vi "controlSensorEnabled.vi"(7 "set":bool, 8 "error in":errorcluster, 9 "enableSensor":bool, 10 "axis":i32, 11 "connection ID":refnum<k5>) -> (0 "error out":errorcluster, 1 "enableSensor out":bool, 2 "axis_out":i32, 3 "connection ID":refnum<k5>)   [LabVIEW 2016, in "AMC_VIs.lvlib"]
doc: "Retrieves or sets sensor power supply status, can be switched off to save heat generated by sensor [NUM or RES]\n Positions retrieved will be invalid when activating this, so closed-loop control should be switched off beforehand."
uses:
  AMC_VIs.lvlib
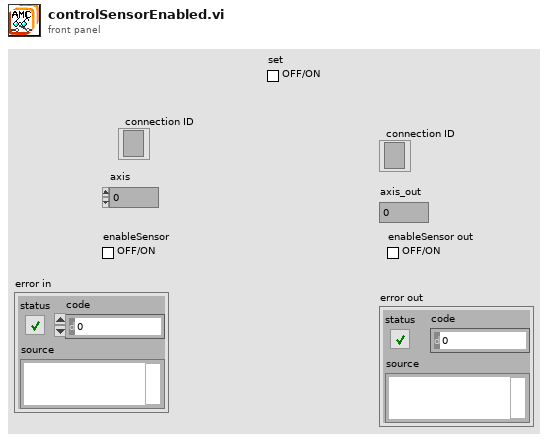
[diagram p1: front panel]
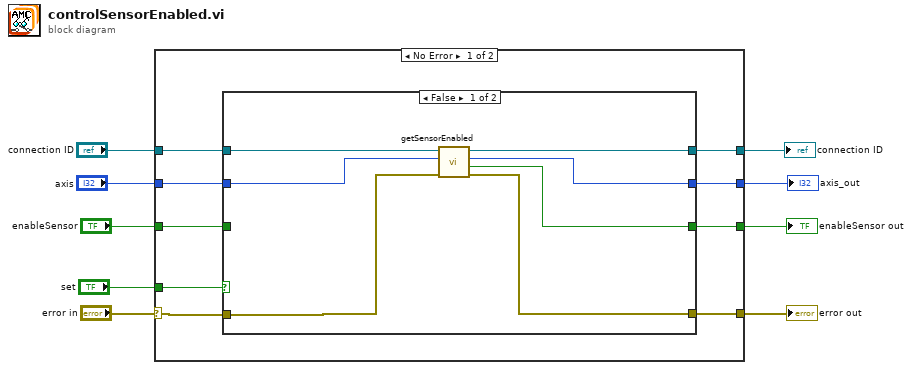
[diagram p0: block diagram]
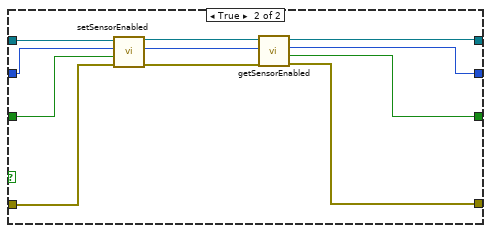
[diagram p2: hidden frame]
diagram:
  n1 = case shown="No Error" "error in" {
    selector: "error in" -> [w16 w40]
    tunnel: [w11 w40] -> w9
    tunnel: [w13 w39] -> w8
    tunnel: "connection ID" -> [w18 w39]
    tunnel: "axis" -> [w15 w37]
    tunnel: "set" -> [w17 _]
    tunnel: "enableSensor" -> [w14 w38]
    tunnel: [w10 w38] -> w2
    tunnel: [w12 w37] -> w1
    frame No Error {
      n2 = case shown="False" w17 {
        tunnel: w18 -> [w25 w36]
        tunnel: w16 -> [w21 w33]
        tunnel: w15 -> [w23 w35]
        tunnel: w14 -> [_ w34]
        tunnel: [w24 w28] -> w13
        tunnel: [w22 w27] -> w12
        tunnel: [w20 w31] -> w11
        tunnel: [w19 w26] -> w10
        frame False {
          n3 = call "getSensorEnabled.vi"("error in"=w21, "axis"=w23, "connection ID"=w25) -> ("error out"=w20:errorcluster, "value"=w19:bool, "axis_out"=w22:i32, "connection ID"=w24:refnum<k5>)  [unwired: 5 in]
        }
        frame True {
          n4 = call "setSensorEnabled.vi"("error in"=w33, "value"=w34, "axis"=w35, "connection ID"=w36) -> ("error out"=w32:errorcluster, "axis_out"=w29:i32, "connection ID"=w30:refnum<k5>)  [unwired: 5 in]
          n5 = call "getSensorEnabled.vi"("error in"=w32, "axis"=w29, "connection ID"=w30) -> ("error out"=w31:errorcluster, "value"=w26:bool, "axis_out"=w27:i32, "connection ID"=w28:refnum<k5>)  [unwired: 5 in]
        }
      }
    }
    frame Error {
    }
  }
  "error out" <- w9
  "connection ID" <- w8
  "axis_out" <- w1
  "enableSensor out" <- w2
